vi "Untitled 4.vi"() -> ()   [LabVIEW 2019]
uses:
  <vilib>/rvi/Emulation/niFpgaGetClockAttributes.vi
  <vilib>/rvi/Emulation/niFpgaSctlEmulationGetInTimedLoop.vi
  <vilib>/rvi/Emulation/niFpgaEmulationReportErrorSimple.vi
  <vilib>/rvi/eio/common/nirviEmuTemplateMethod_errors.vi
  <vilib>/rvi/Emulation/niFpgaCriticalErrorInLSC.vi
  <vilib>/eio/EIONode/EIONode.xnode
panel:
  out "x-y":u32
  out "Count":i32
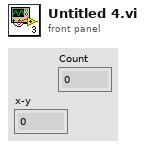
[diagram p1: front panel]
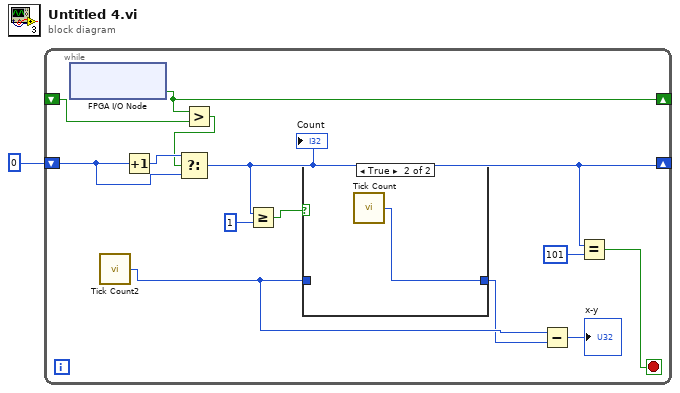
[diagram p0: block diagram]
diagram:
  n1 = while {
    shift-right: [w14] -> _
    shift-left: _ -> [w13]
    shift-right: [w4] -> _
    shift-left: 0 ("x") -> [w11]
    stop <- w2 stop-if-true
    n2 = xnode "FPGA I/O Node"() -> ("Mod8/DI1"=w14:bool)  [unwired: 1 in, 1 out]
    n3 = call "Tick Count2"() -> ("Tick Count(mSec)"=w9:u32)
    n4 = Increment(x=w11) -> (x+1=w12:i32)
    n5 = Greater?(x=w14, y=w13) -> (0:w10:bool)
    n6 = Select(t=w12, s=w10, f=w11) -> (s? t:f=w4:i32)
    "Count" <- w4
    n7 = Greater Or Equal?(x=w4, y=1) -> (x >= y?=w5:bool)
    n8 = case shown="True" w5 {
      tunnel: [w15 w16] -> w8
      tunnel: w9 -> [w15 _]
      frame False {
      }
      frame True {
        n9 = call "Tick Count"() -> ("Tick Count(mSec)"=w16:u32)
      }
    }
    n10 = Subtract(x=w9, y=w8) -> (x-y=→"x-y":u32)
    n11 = Equal?(x=w4, y=101) -> (x = y?=w2:bool)
  }
